vi "Read R.vi"(8 "error in (no error)":errorcluster, 11 "Ball in":refnum<class "Ball.lvclass">) -> (0 "error out":errorcluster, 2 "Real Matrix":T1, 3 "Ball out":refnum<class "Ball.lvclass">)   [LabVIEW 2018, in "Ball.lvclass"]
uses:
  Ball.lvclass
  <vilib>/Analysis/Matrix/Datatypes/RealMatrix.ctl
  Ball.lvclass/Ball.ctl
  <vilib>/Analysis/Matrix/NI_Matrix.lvlib
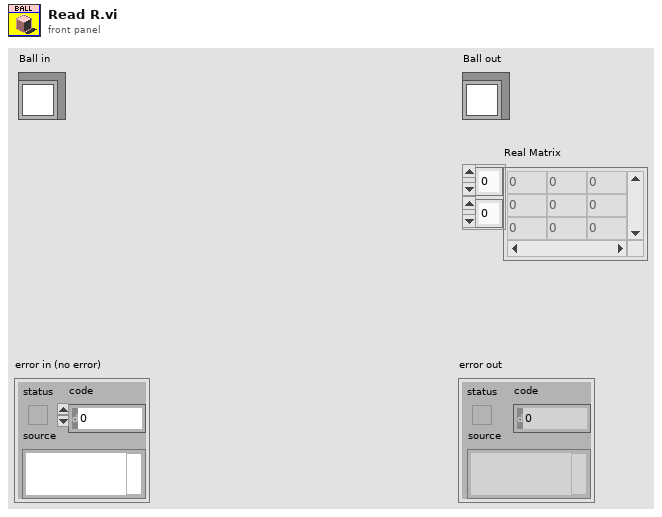
[diagram p1: front panel]
types:
  T1 = typedef "NI_Matrix.lvlib/RealMatrix.ctl" = dbl[][]
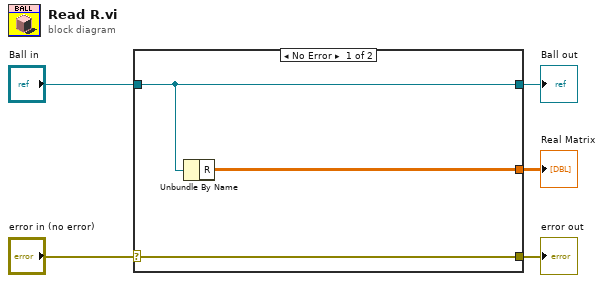
[diagram p0: block diagram]
diagram:
  n1 = case shown="No Error" "error in (no error)" {
    selector: "error in (no error)" -> [w8 w9]
    tunnel: [w8 w9] -> w4
    tunnel: [w7 w10] -> w2
    tunnel: "Ball in" -> [w7 w10]
    tunnel: [w6 _] -> w1
    frame No Error {
      n2 = Unbundle By Name(w7) -> ("R"=w6:T1)
    }
    frame Error {
    }
  }
  "error out" <- w4
  "Ball out" <- w2
  "Real Matrix" <- w1
